vi "ECS - System - User Interface Calpoints.vi"   [LabVIEW 2015, in "ECS-RT.lvlib"]
uses:
  ECS-RT.lvlib
  Globals/Calpoint IDs.vi
  <vilib>/addons/Software Calibration Management/_CalPointResources/scm32.dll
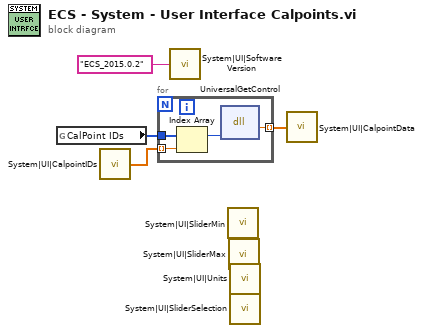
[diagram p0: block diagram]
diagram:
  n1 = global read "Calpoint IDs.vi" "CalPoint IDs"() -> (w4:i32[])
  n2 = call "System|UI|CalpointIDs"() -> ("Value"=w3:sgl[])
  n3 = for {
    tunnel: w4 -> [w8]
    tunnel: [w7] -> w2 mode=indexing
    tunnel: w3 -> [w5] mode=indexing
    n4 = Index Array(array=w8, index=w5) -> (element=w6:i32)
    n5 = dll-call lib="C:/Program Files (x86)/National Instruments/LabVIEW 2015/vi.lib/addons/Software Calibration Management/_CalPointResources/scm*.*" fn="UniversalGetControl"("ID"=w6) -> ("return type"=w7:sgl)  [unwired: 4 in, 2 out]
  }
  n6 = call "System|UI|Software Version"("Value"="ECS_2015.0.2") -> ()
  n7 = call "System|UI|SliderMin"() -> ()  [unwired: 1 out]
  n8 = call "System|UI|SliderMax"() -> ()  [unwired: 1 out]
  n9 = call "System|UI|Units"() -> ()  [unwired: 1 out]
  n10 = call "System|UI|SliderSelection"() -> ()  [unwired: 1 out]
  n11 = call "System|UI|CalpointData"("Value"=w2) -> ()
